vi "Configure Memory and Time.vi"(8 "error in (no error)":errorcluster, 9 "Memory Location (000)":i32 min=0 max=399 step=1 format="%03.0f", 10 "Dispense Time (0000)":i64 min=0 max=99999 step=1 format="%05.0f", 11 "VISA resource name":refnum<visa-resource-name>) -> (0 "error out":errorcluster, 3 "VISA resource name out":refnum<visa-resource-name>)   [LabVIEW 2020, in "EFD Ultimus V.lvlib"]
doc: "Updates the dispense time value in the memory location specified in the command. This command will update the LCD screen to the specified memory location.\n\nHost Format: DH--CHcccTttttt\n ccc:The 3 digit memory location from 0-399.\n ttttt:The four or five digit dispense time value excluding the decimal point. The valid range is 0.0000 to \n 9.9999. This command for this VI only accepts 4 decimal places."
uses:
  EFD Ultimus V.lvlib
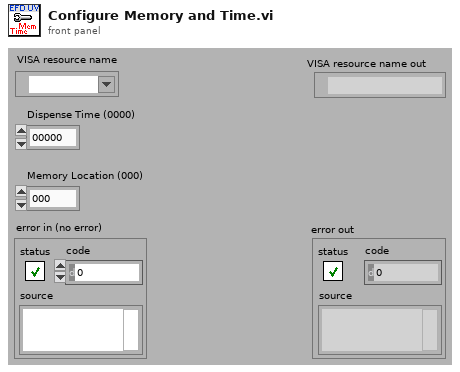
[diagram p1: front panel]
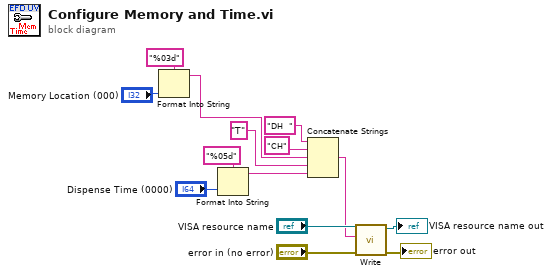
[diagram p0: block diagram]
diagram:
  n1 = Format Into String(format string="%03d", "Memory Location (000)") -> (resulting string=w6:string)  [unwired: 2 in, 1 out]
  n2 = Format Into String(format string="%05d", "Dispense Time (0000)") -> (resulting string=w3:string)  [unwired: 2 in, 1 out]
  n3 = Concatenate Strings("DH  " ("string"), "CH" ("string"), w6, "T" ("string"), w3) -> (w9:string)
  n4 = call "Write.vi"("error in (no error)"="error in (no error)", "Command To Write"=w9, "VISA resource name"="VISA resource name") -> ("error out"=→"error out":errorcluster, "VISA resource name out"=→"VISA resource name out":refnum<visa-resource-name>)  [unwired: 7 out]
